vi "Calcu_Standard Pressure.vi"(0 "λ":dbl, 1 "A0":dbl, 3 "Ts":dbl, 4 "ρa":dbl, 5 "σ":dbl, 6 "M":dbl[](array[numeric]), 8 "Ta":dbl, 9 "P":dbl) -> (7 "결과":dbl)   [LabVIEW 2020]
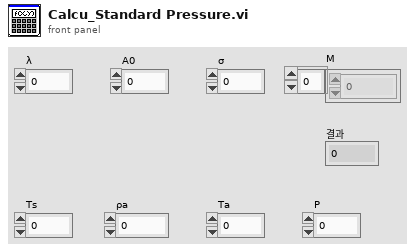
[diagram p1: front panel]
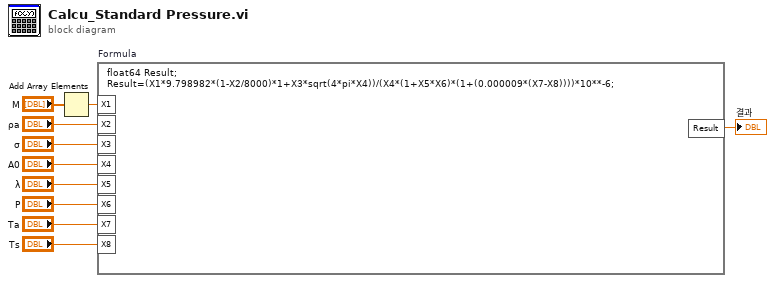
[diagram p0: block diagram]
diagram:
  n1 = Add Array Elements(numeric array="M") -> (sum=w1:dbl)
  n2 = formula code="float64 Result;\nResult=(X1*9.798982*(1-X2/8000)*1+X3*sqrt(4*pi*X4))/(X4*(1+X5*X6)*(1+(0.000009*(X7-X8))))*10**-6;"("X1"=w1, "X2"="ρa", "X3"="σ", "X4"="A0", "X5"="λ", "X6"="P", "X7"="Ta", "X8"="Ts") -> ("Result"=→"결과":dbl)
